vi "Configure Math Channel FFT.vi"(6 "FFT Vertical Scale (dBV RMS)":string(combo)="LOGRMS", 8 "error in (no error)":errorcluster {"code" format="%.0x"}, 9 "FFT Window (Rectangular)":string(combo)="RECTANGULAR", 10 "Math Source (CH1)":string(combo)="CH1", 11 "VISA Resource Name":refnum<visa-resource-name>) -> (0 "error out":errorcluster {"code" format="%.0x"}, 3 "VISA Resource Name Out":refnum<visa-resource-name>)   [LabVIEW 2010, in "Tektronix TDS 3000 Series.lvlib"]
doc: "This VI configures a math channel to calculate an FFT."
uses:
  <instrlib>/Tektronix TDS 3000 Series/Tektronix TDS 3000 Series.lvlib
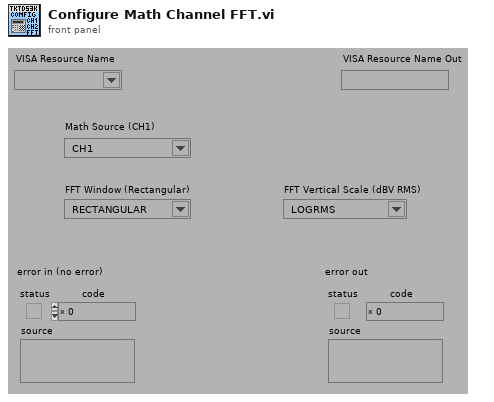
[diagram p1: front panel]
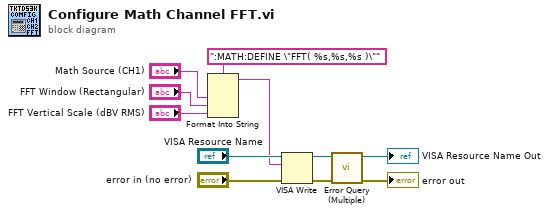
[diagram p0: block diagram]
diagram:
  n1 = Format Into String(format string=":MATH:DEFINE \"FFT( %s,%s,%s )\"", "Math Source (CH1)", "FFT Window (Rectangular)", "FFT Vertical Scale (dBV RMS)") -> (resulting string=w5:string)  [unwired: 2 in, 1 out]
  n2 = VISA Write(VISA resource name="VISA Resource Name", write buffer=w5, error in (no error)="error in (no error)") -> (VISA resource name out=w4:refnum<visa-resource-name>, error out=w3:errorcluster)  [unwired: 1 out]
  n3 = call <instrlib>:"Error Query (Multiple).vi"("error in (no error)"=w3, "VISA Resource Name"=w4) -> ("error out"=→"error out":errorcluster, "VISA Resource Name Out"=→"VISA Resource Name Out":refnum<visa-resource-name>)  [unwired: 6 in, 2 out]
